vi "XIPIN_UltraScale_Soft_Error_Mitigation_3_0.vi"   [LabVIEW 2017]
doc: "The Xilinx Soft Error Mitigation IP solution provides a pre-verified design which can detect and optionally correct and classify soft errors in Configuration Memory. A soft error is an unintended change to the state of memory bits caused by ionizing radiation. The solution does not prevent soft errors; rather, it provides users with a method to better manage the system-level effects of these events. Intelligent management of these events can increase reliability and availability, and reduce system maintenance and downtime costs. This Soft Error Mitigation IP is for the UltraScale FPGAs and newer architectures.\n------------------------------------\n<b>Need License</b> : No"
uses:
  <vilib>/rvi/XilinxIP/XIPIN_XNode/niFpgaXIPIN.xnode
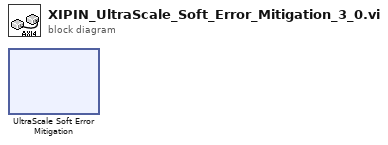
[diagram p0: block diagram]
diagram:
  n1 = xnode ("UltraScale Soft Error Mitigation")() -> ()
